vi "Default Path.vi"(8 "error in (no error)":errorcluster, 10 "Folder Name":string="Configuration.ini", 11 "Configuration in":refnum<class "Configuration.lvclass">) -> (0 "error out":errorcluster, 3 "Configuration out":refnum<class "Configuration.lvclass">)   [LabVIEW 2019, in "Configuration.lvclass"]
uses:
  Configuration.lvclass
  <vilib>/Utility/sysdir.llb/System Directory Type.ctl
  Configuration.lvclass/Configuration.ctl
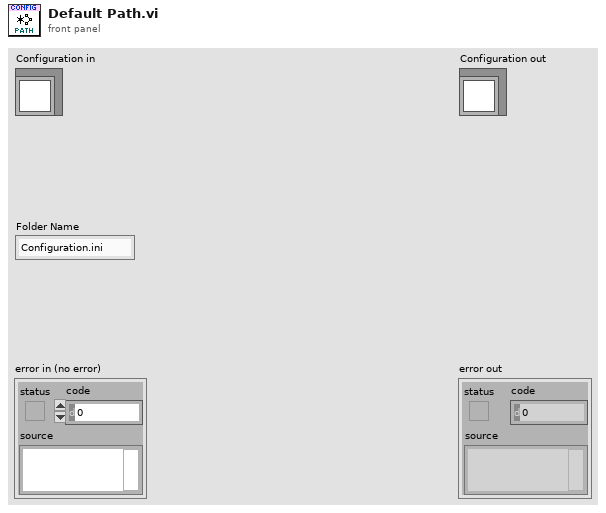
[diagram p1: front panel]
types:
  T1 = typedef "System Directory Type.ctl" = i32
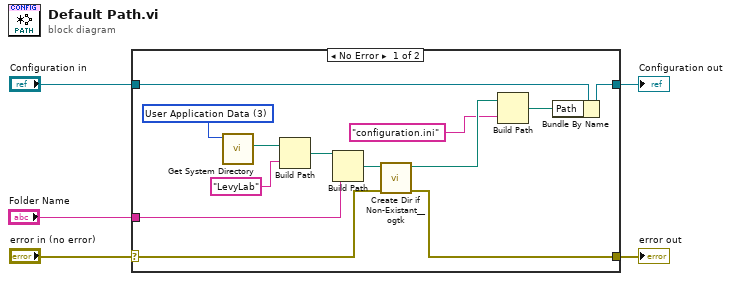
[diagram p0: block diagram]
diagram:
  n1 = case shown="No Error" "error in (no error)" {
    selector: "error in (no error)" -> [w8 w19]
    tunnel: [w7 w19] -> w4
    tunnel: [w17 w20] -> w2
    tunnel: "Configuration in" -> [w18 w20]
    tunnel: "Folder Name" -> [w9 _]
    frame No Error {
      w14 = T1 3 items=["User Home"=0, "User Desktop"=1, "User Documents"=2, "User Application Data"=3, "User Preferences"=4, "User Temporary"=5, "Public Documents"=6, "Public Application Data"=7, "Public Preferences"=8, "Public Cache"=13, "System Core Libraries"=9, "System Installed Libraries"=10, "Application Files"=11, "Boot Volume Root"=12] ("system directory type")
      n2 = call <vilib>:"Get System Directory.vi"("system directory type"=w14) -> ("system directory"=w13:path)  [unwired: 10 in]
      n3 = Build Path(base path=w13, name or relative path="LevyLab") -> (appended path=w11:path)
      n4 = Build Path(base path=w11, name or relative path=w9) -> (appended path=w15:path)
      n5 = call <userlib>:"Create Dir if Non-Existant__ogtk.vi"("error in (no error)"=w8, "Directory Path"=w15) -> ("error out"=w7:errorcluster, "dup Directory Path"=w16:path)  [unwired: 7 in, 1 out]
      n6 = Build Path(base path=w16, name or relative path="configuration.ini") -> (appended path=w10:path)
      n7 = Bundle By Name(cluster=w18, "Path"=w10) -> (w17:refnum<class "Configuration.lvclass">)
    }
    frame Error {
    }
  }
  "error out" <- w4
  "Configuration out" <- w2
